vi "update channel names to match tags.vi"(8 "error in":errorcluster, 10 "TEC in":refnum<class "TEC configuration.lvclass">, 11 "engine configuration in":refnum<class "engine configuration.lvclass">) -> (0 "error out":errorcluster, 2 "TEC out":refnum<class "TEC configuration.lvclass">, 3 "engine configuration out":refnum<class "engine configuration.lvclass">)   [LabVIEW 2013, in "TEC editor node.lvclass"]
uses:
  TEC editor node.lvclass
  module/configuration/TEC configuration.lvclass
  <vilib>/NI/Module Execution Interface/Engine Configuration/engine configuration.lvclass
  <vilib>/NI/Configuration Framework/serializable configuration/NISE_CEF_serializable configuration.lvclass/NISE_CEF_serializable configuration.ctl
  <vilib>/NI/Configuration Framework/serializable configuration/NISE_CEF_serializable configuration.lvclass
  module/configuration/TEC configuration.lvclass/TEC configuration.ctl
  <vilib>/NI/Tag Bus/tag/tag descriptor.lvclass/tag descriptor.ctl
  <vilib>/NI/Tag Bus/tag/read tag name.vi
  <vilib>/NI/Configuration Framework/serializable configuration/Read UID.vi
  module/configuration/Read channels.vi
  <vilib>/NI/Tag Bus Module Framework/channel/TBM channel.lvclass
  <vilib>/NI/Tag Bus/tag/tag descriptor.lvclass
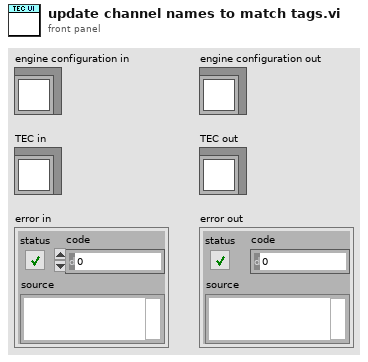
[diagram p1: front panel]
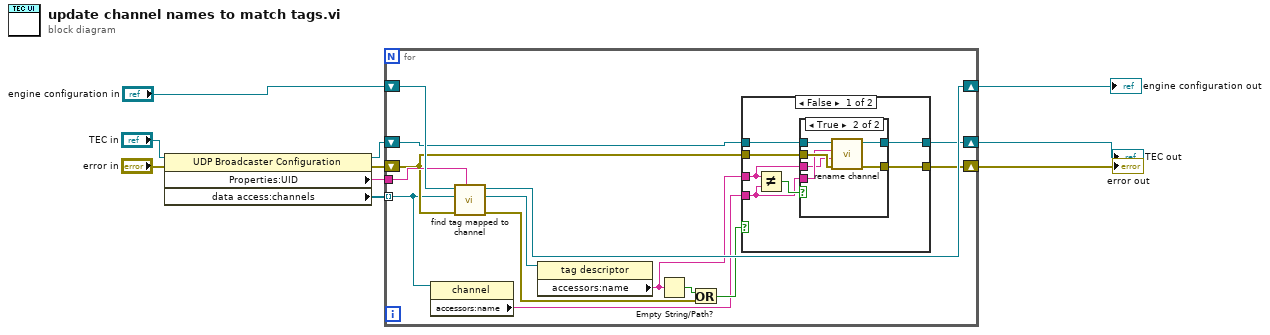
[diagram p0: block diagram]
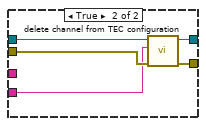
[diagram p3: hidden frame]
diagram:
  n1 = property class="UDP Broadcaster Configuration"(reference="TEC in", error in="error in") -> (reference out=w3:refnum<class "TEC configuration.lvclass">, error out=w2:errorcluster, "Properties:UID"=w6:string, "data access:channels"=w1:refnum<class "TBM channel.lvclass">[])
  n2 = for {
    tunnel: w1 -> [w14] mode=indexing
    shift-right: [w22] -> w7
    shift-left: "engine configuration in" -> [w24]
    shift-right: [w19] -> w4
    shift-left: w3 -> [w17]
    tunnel: w6 -> [w23]
    shift-right: [w18] -> w5
    shift-left: w2 -> [w15]
    n3 = property class="channel"(reference=w14) -> ("accessors:name"=w12:string)  [unwired: 1 in, 2 out]
    n4 = call <vilib>:"find tag mapped to channel.vi"("owner"=w23, "error in"=w15, "channel"=w14, "engine configuration in"=w24) -> ("error out"=w13:errorcluster, "tag"=w21:refnum<class "tag descriptor.lvclass">, "engine configuration out"=w22:refnum<class "engine configuration.lvclass">)  [unwired: 5 in]
    n5 = property class="tag descriptor"(reference=w21) -> ("accessors:name"=w11:string)  [unwired: 1 in, 2 out]
    n6 = Empty String/Path?(string/path=w11) -> (empty?=w20:bool)
    n7 = Or(x=w20, y=w13) -> (x .or. y?=w16:bool)
    n8 = case shown="False" w16 {
      tunnel: [w28 w44] -> w19
      tunnel: [w31 w43] -> w18
      tunnel: w15 -> [w30 w42]
      tunnel: w17 -> [w29 w41]
      tunnel: w12 -> [w26 w40]
      tunnel: w11 -> [w25 _]
      frame False {
        n9 = Not Equal?(x=w25, y=w26) -> (x != y?=w27:bool)
        n10 = case shown="True" w27 {
          tunnel: [w33 w38] -> w31
          tunnel: w30 -> [w33 w39]
          tunnel: w29 -> [w32 w37]
          tunnel: [w32 w36] -> w28
          tunnel: w26 -> [_ w35]
          tunnel: w25 -> [_ w34]
          frame False {
          }
          frame True {
            n11 = call "rename channel.vi"("error in"=w39, "new name"=w34, "old name"=w35, "TEC configuration in"=w37) -> ("error out"=w38:errorcluster, "TEC configuration out"=w36:refnum<class "TEC configuration.lvclass">)  [unwired: 6 in]
          }
        }
      }
      frame True {
        n12 = call "delete channel from TEC configuration.vi"("error in"=w42, "channel to delete"=w40, "TEC configuration in"=w41) -> ("error out"=w43:errorcluster, "TEC configuration out"=w44:refnum<class "TEC configuration.lvclass">)  [unwired: 7 in]
      }
    }
  }
  "engine configuration out" <- w7
  "error out" <- w5
  "TEC out" <- w4
